vi "Test OrderSelection.vi"() -> ()   [LabVIEW 2015, in "OrderSelection.lvclass"]
uses:
  OrderSelection.lvclass
  <vilib>/Utility/miscctls.llb/LVPointTypeDef.ctl
  Write Items.vi
  Read Items.vi
panel:
  out "Items[]":string[](array[string])
  out "Selector":picture
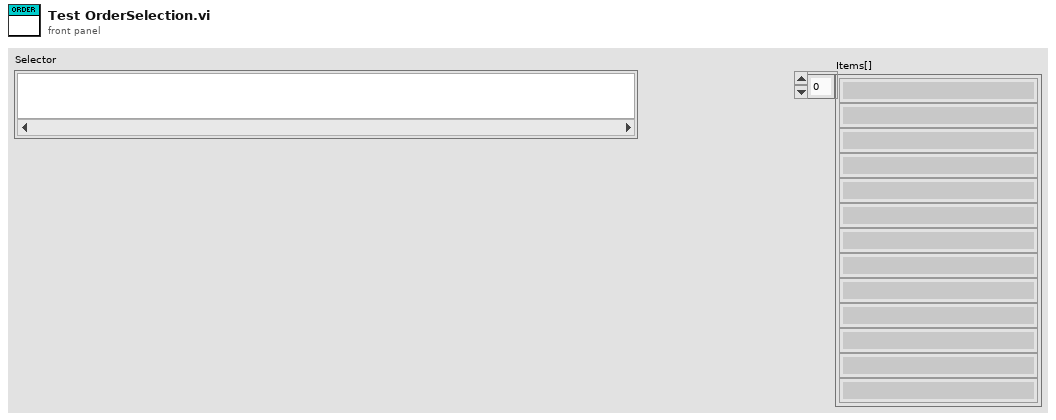
[diagram p1: front panel]
types:
  T1 = typedef "LVPointTypeDef.ctl" = cluster{"Horizontal":i16, "Vertical":i16}
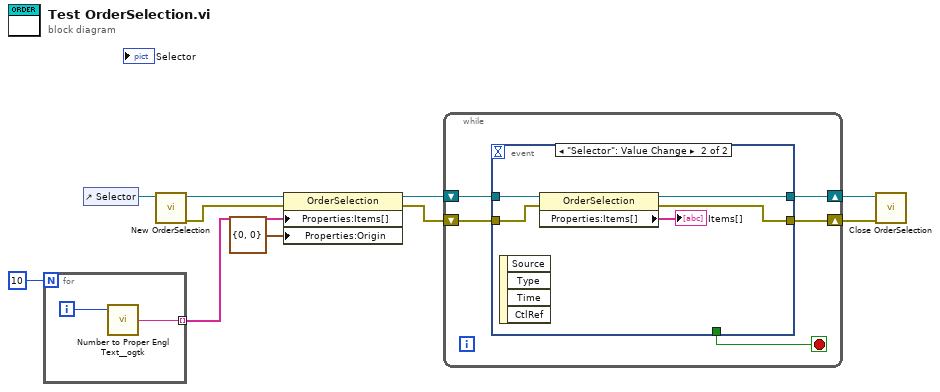
[diagram p0: block diagram]
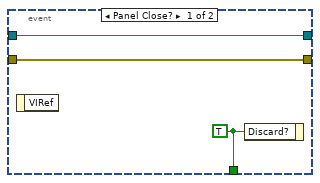
[diagram p2: hidden frame]
diagram:
  n1 = for {
    N: 10 -> [_]
    tunnel: [w11] -> w2 mode=indexing
    i -> [w12]
    n2 = call <userlib>:"Number to Proper Engl Text__ogtk.vi"("Numeric"=w12) -> ("String"=w11:string)  [unwired: 4 in]
  }
  n3 = control-ref of="Selector"() -> (w7:refnum<vi>)
  n4 = call "New OrderSelection.vi"("Reference"=w7) -> ("error out"=w9:errorcluster, "OrderSelection out"=w5:refnum<class "OrderSelection.lvclass">)  [unwired: 9 in]
  n5 = property class="OrderSelection"(reference=w5, error in=w9, "Properties:Items[]"=w2, "Properties:Origin"=T1 {"Horizontal"=0, "Vertical"=0} ("Origin: All Elements")) -> (reference out=w4:refnum<class "OrderSelection.lvclass">, error out=w6:errorcluster)
  n6 = while {
    shift-right: [w16] -> w10
    shift-left: w4 -> [w15]
    shift-right: [w14] -> w8
    shift-left: w6 -> [w13]
    stop <- w17 stop-if-true
    n7 = event shown="[1] \"Selector\": Value Change" {
      selector: _ -> [_ _]
      dyn-events: _ -> [_ _]
      timeout: _ -> [_ _]
      tunnel: [w20 _] -> w17
      tunnel: [w19 w24] -> w16
      tunnel: w15 -> [w19 w25]
      tunnel: [w18 w21] -> w14
      tunnel: w13 -> [w18 w22]
      event Panel Close? {
        w20 = TRUE ("Discard?")
        n8 = event-data() -> ()  [unwired: 1 in, 1 out]
        n9 = event-data("Discard?"=w20) -> ()  [unwired: 1 in, 1 out]
      }
      event "Selector": Value Change {
        n10 = event-data() -> ()  [unwired: 1 in, 4 out]
        n11 = property class="OrderSelection"(reference=w25, error in=w22) -> (reference out=w24:refnum<class "OrderSelection.lvclass">, error out=w21:errorcluster, "Properties:Items[]"=→"Items[]":string[])
      }
    }
  }
  n12 = call "Close OrderSelection.vi"("error in (no error)"=w8, "OrderSelection in"=w10) -> ()  [unwired: 9 in, 1 out]
